vi "Lift control.vi"(10 "Lift button?":bool, 11 "Lift Current":dbl) -> (3 "Lift power":dbl format="%#_13g")   [LabVIEW 2016]
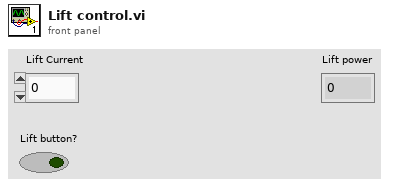
[diagram p1: front panel]
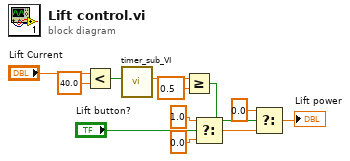
[diagram p0: block diagram]
diagram:
  n1 = Less?(x="Lift Current", y=40.0) -> (x < y?=w1:bool)
  n2 = call "timer_sub_VI.vi"("Reset"=w1) -> ("Time (Secs)"=w9:dbl)  [unwired: 10 in]
  n3 = Greater Or Equal?(x=w9, y=0.5) -> (x >= y?=w6:bool)
  n4 = Select(t=1.0, s="Lift button?", f=0.0) -> (s? t:f=w7:dbl)
  n5 = Select(t=0.0, s=w6, f=w7) -> (s? t:f=→"Lift power":dbl)
